vi "Open and Close-VI.vi"(0 "State":T1(ring)=enum."Standard", 1 "Close VI":path, 11 "error in":errorcluster, 12 "Open VI":path) -> (15 "error out":errorcluster)   [LabVIEW 2019]
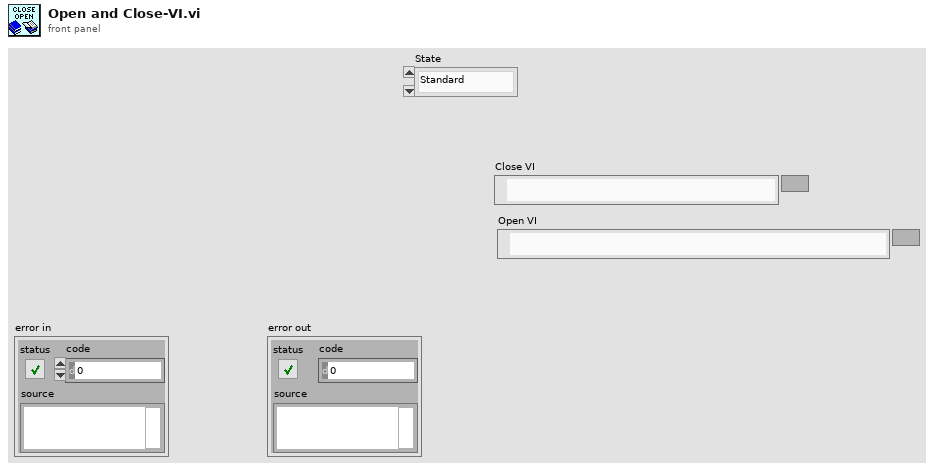
[diagram p1: front panel]
types:
  T1 = enum32{"Invalid", "Standard", "Closed", "Hidden", "Minimized", "Maximized"}
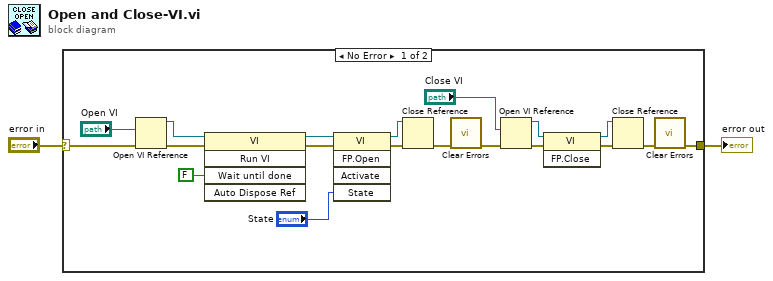
[diagram p0: block diagram]
diagram:
  n1 = case shown="No Error" "error in" {
    selector: "error in" -> [w13 w22]
    tunnel: [w12 w22] -> w2
    frame No Error {
      n2 = Open VI Reference(vi path="Open VI", error in (no error)=w13) -> (vi reference=w4:refnum<vi>, error out=w3:errorcluster)  [unwired: 4 in]
      n3 = invoke class="VI" method="Run VI"(reference=w4, error in=w3, "Wait until done"=FALSE ("Wait Until Done")) -> (reference out=w6:refnum<vi>, error out=w7:errorcluster)  [unwired: 2 in, 3 out]
      n4 = invoke class="VI" method="FP.Open"(reference=w6, error in=w7, "State"="State") -> (reference out=w10:refnum<vi>, error out=w9:errorcluster)  [unwired: 2 in, 3 out]
      n5 = Close Reference(reference=w10, error in (no error)=w9) -> (error out=w16:errorcluster)
      n6 = call <vilib>:"Clear Errors.vi"("error in (no error)"=w16) -> ("error out"=w15:errorcluster)  [unwired: 5 in, 1 out]
      n7 = Open VI Reference(vi path="Close VI", error in (no error)=w15) -> (vi reference=w21:refnum<vi>, error out=w14:errorcluster)  [unwired: 4 in]
      n8 = invoke class="VI" method="FP.Close"(reference=w21, error in=w14) -> (reference out=w18:refnum<vi>, error out=w19:errorcluster)  [unwired: 1 in, 1 out]
      n9 = Close Reference(reference=w18, error in (no error)=w19) -> (error out=w17:errorcluster)
      n10 = call <vilib>:"Clear Errors.vi"("error in (no error)"=w17) -> ("error out"=w12:errorcluster)  [unwired: 5 in, 1 out]
    }
    frame Error {
    }
  }
  "error out" <- w2
